vi "save settings.vi"(8 "error in (no error)":errorcluster, 11 "Type Signal":T1={"DAQ Board Name"="DAQ_Simu1", "Analogicos Canales"=["DAQ_Simu1/ai1", "DAQ_Simu1/ai2"], "rate"=1000.0, "number of samples "=1000, "Tiempo"=100}) -> (0 "error out":errorcluster)   [LabVIEW 2020, in "Settings.lvlib"]
uses:
  Settings.lvlib
  typeSignal--cluster.ctl
  <vilib>/drjdpowell/SQLite Library/SQL Connection/Open (path).vi
  <vilib>/drjdpowell/SQLite Library/SQL Connection/Open (string).vi
  <vilib>/AdvancedString/Path To Command Line String.vi
  <vilib>/drjdpowell/SQLite Library/SQL Connection/Execute SQL (No results).vi
  <vilib>/drjdpowell/SQLite Library/SQL Connection/Connection.lvclass
  <vilib>/drjdpowell/SQLite Library/SQLite.lvlib
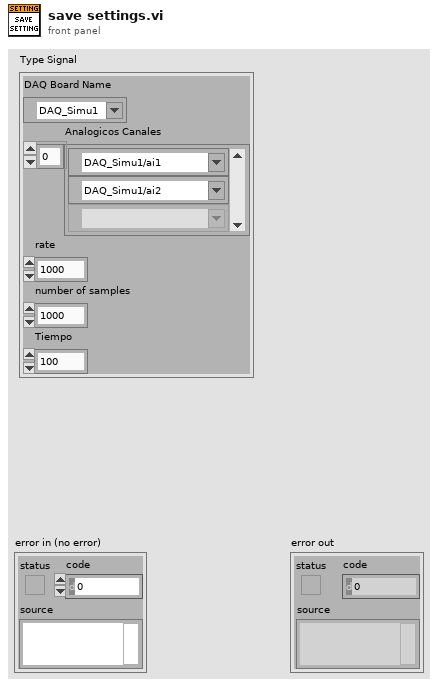
[diagram p1: front panel]
types:
  T1 = typedef "typeSignal--cluster.ctl" = cluster{"DAQ Board Name":tag, "Analogicos Canales":tag[], "rate":dbl, "number of samples ":i32, "Tiempo":i32}
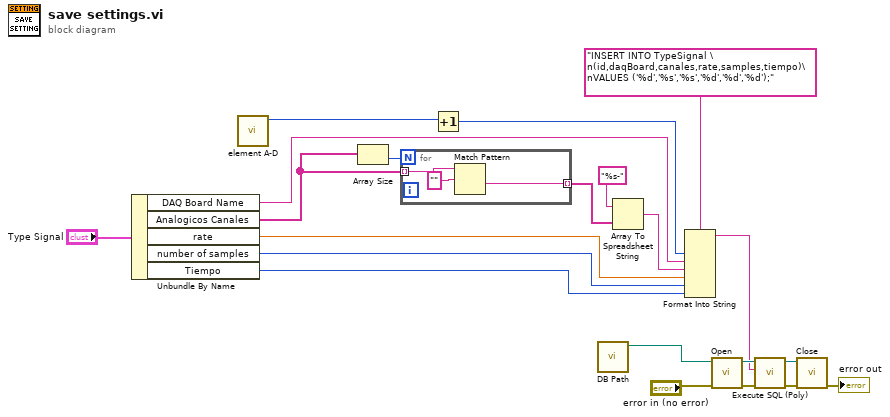
[diagram p0: block diagram]
diagram:
  n1 = Unbundle By Name("Type Signal") -> ("DAQ Board Name"=w14:tag, "Analogicos Canales"=w9:tag[], "rate"=w4:dbl, "number of samples"=w3:i32, "Tiempo"=w2:i32)
  n2 = call "element A-D.vi"() -> ("max(x,y)"=w1:i64)  [unwired: 10 in, 1 out]
  n3 = Array Size(array=w9) -> (size(s)=w12:i32)
  n4 = for {
    N: w12 -> [_]
    tunnel: w9 -> [w24] mode=indexing
    tunnel: [w22] -> w11 mode=indexing
    n5 = Match Pattern(string=w24, regular expression="") -> (after substring=w22:string)  [unwired: 1 in, 3 out]
  }
  n6 = Increment(x=w1) -> (x+1=w5:i64)
  n7 = call "DB Path.vi"() -> ("DB path"=w7:path)  [unwired: 11 in]
  n8 = Array To Spreadsheet String(array=w11, 3:"%s-" ("delimiter (Tab)")) -> (spreadsheet string=w8:string)  [unwired: 1 in]
  n9 = Format Into String(format string="INSERT INTO TypeSignal \n(id,daqBoard,canales,rate,samples,tiempo)\nVALUES ('%d','%s','%s','%d','%d','%d');", w5, w14, w8, w4, w3, w2) -> (resulting string=w13:string)  [unwired: 2 in, 1 out]
  n10 = call-poly <vilib>:"Open.vi"("error in (no error)"="error in (no error)", "db file"=w7) -> ("error out"=w21:errorcluster, "SQLite Connection"=w20:refnum<class "Connection.lvclass">)  [unwired: 8 in]
  n11 = call-poly <vilib>:"Execute SQL (Poly).vi"("error in (no error)"=w21, "SQL"=w13, "SQLite Connection in"=w20) -> ("error out"=w18:errorcluster, "SQLite Connection"=w19:refnum<class "Connection.lvclass">)  [unwired: 7 in]
  n12 = call-dynamic "Close.vi"("error in (no error)"=w18, "SQLite Connection in"=w19) -> ("error out"=→"error out":errorcluster)  [unwired: 9 in]
